vi "Sensado_mioelectrico_Final.vi"() -> ()   [LabVIEW 2010]
uses:
  <vilib>/express/express analysis/Spectral/XNode/ExpressSpectralMeasurementsBlockNode.xnode
  <vilib>/express/express analysis/Spectral/Block/exnSpectralBlock spectral measurements RMS poly.vi
  <vilib>/express/express analysis/Spectral/Block/exnSpectralBlock spectral measurements RMS WFM.vi
  <vilib>/measure/NI_MABase.lvlib
  <vilib>/express/express analysis/Spectral/Block/exnSpectralBlock spectral measurements power poly.vi
  <vilib>/express/express analysis/Spectral/Block/exnSpectralBlock spectral measurements power WFM.vi
  <vilib>/express/express analysis/Spectral/Block/exnSpectralBlock spectral measurements PSD poly.vi
  <vilib>/express/express analysis/Spectral/Block/exnSpectralBlock spectral measurements PSD WFM.vi
panel:
  in  "Lesion Off\nLesion On":bool
  out "Frecuencia normal":bool
  out "Persona Sana":bool
  out "Señal Anormal":bool
  out "Fatiga":bool
  out "Frecuencia promedio":dbl
  out "Voltaje RMS":dbl format="%0.2f"
  out "Tiempo s":u32
  out "SEMG Filtrada":waveform(dbl)(graph)
  out "FFT sin Filtrado":cluster{"f0":dbl, "df":dbl, "magnitude":dbl[]}(graph) caption="Filtered Signal"
  out "DDT Power Spectrum Density":cluster{"f0":dbl, "df":dbl, "magnitude":dbl[]}(graph) caption="Filtered Signal"
  out "Power Spectrum":cluster{"f0":dbl, "df":dbl, "magnitude":dbl[]}(graph) caption="Filtered Signal"
  out "FFT Filtrada":cluster{"f0":dbl, "df":dbl, "magnitude":dbl[]}(graph) caption="Filtered Signal"
  out "SEMG Bruto":waveform(dbl)(graph)
  in  "Stop":bool
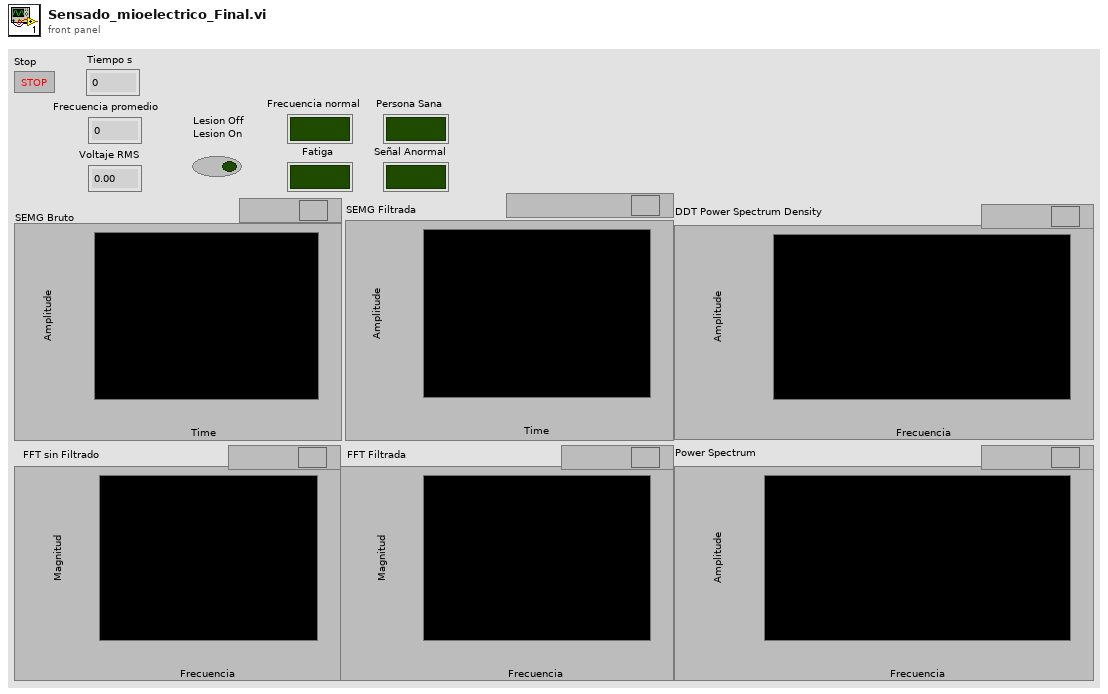
[diagram p1: front panel]
types:
  T1 = enum16{"Sine Wave", "Triangle Wave", "Square Wave", "Sawtooth Wave"}
  T2 = cluster{"averaging mode":u16, "weighting mode":u16, "number of averages":u32}
  T3 = cluster{"dB On (F)":bool, "unwrap phase (F)":bool, "convert to degree (F)":bool}
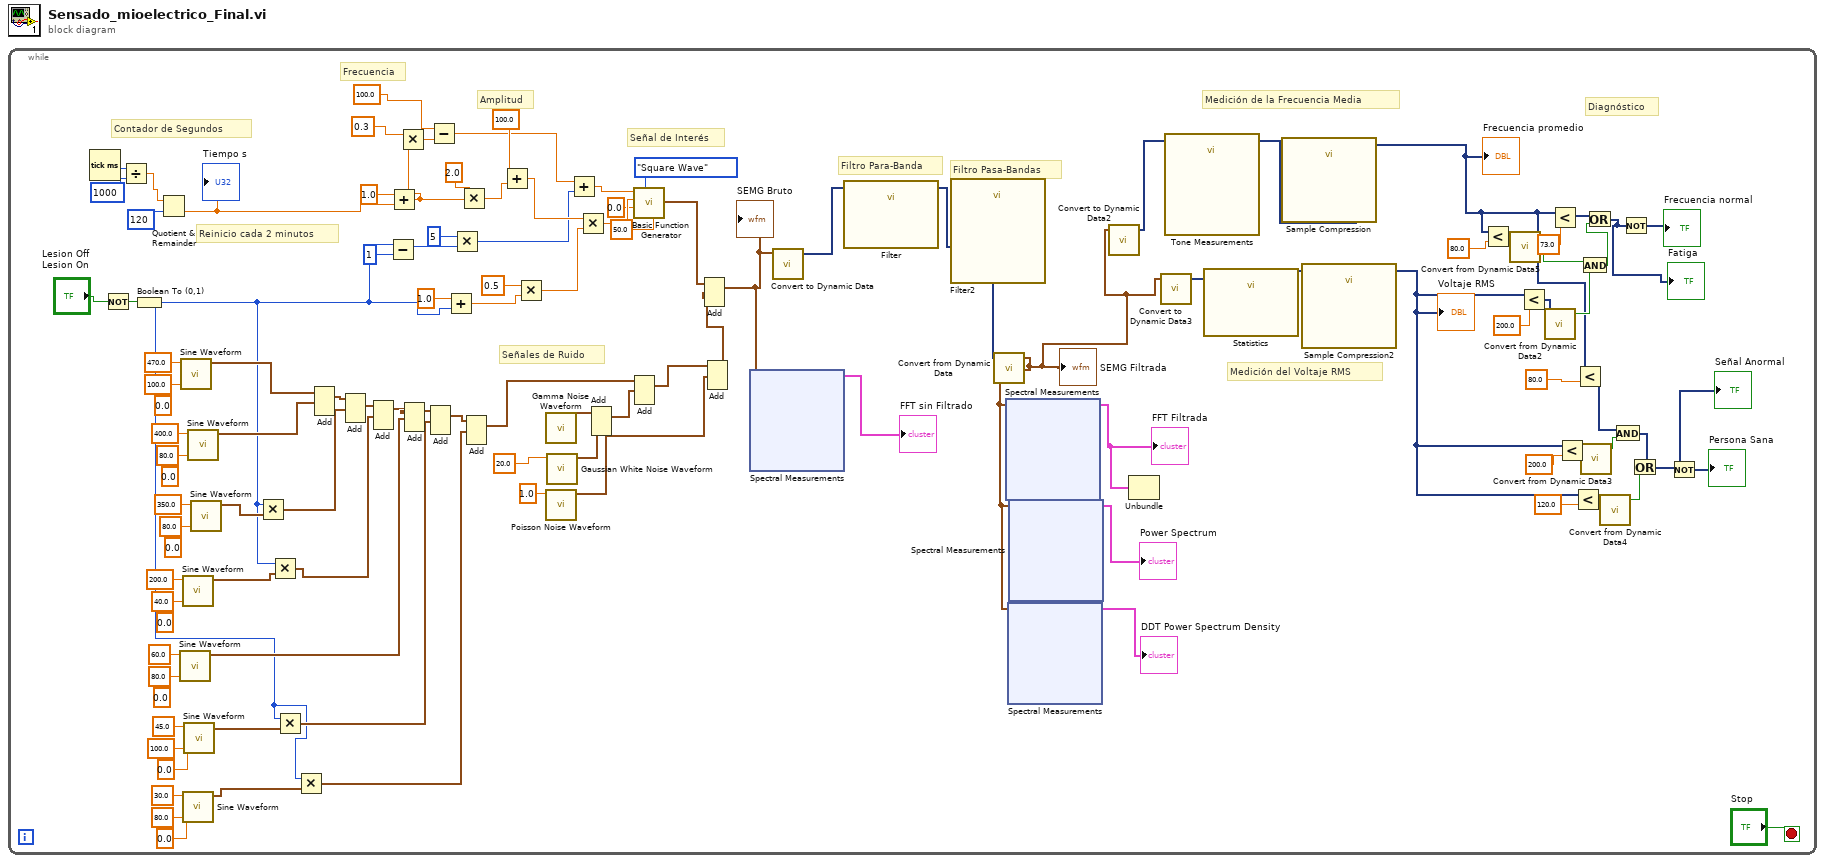
[diagram p0: block diagram]
diagram:
  n1 = while {
    stop <- "Stop" stop-if-true
    (unwired) 0.0 ("phase")
    (unwired) 0.0 ("phase")
    (unwired) 0.0 ("phase")
    (unwired) 0.0 ("phase")
    (unwired) 0.0 ("phase")
    # "Señal de Interés"
    # "Diagnóstico"
    # "Medición del Voltaje RMS"
    # "Medición de la Frecuencia Media"
    # "Filtro Pasa-Bandas"
    # "Filtro Para-Banda"
    # "Señales de Ruido"
    # "Reinicio cada 2 minutos"
    # "Contador de Segundos"
    # "Amplitud"
    # "Frecuencia"
    n2 = Tick Count (ms)() -> (millisecond timer value=w69:u32)
    n3 = Not(x="Lesion Off\nLesion On") -> (.not. x?=w37:bool)
    n4 = Divide(x=w69, y=u32 1000) -> (x/y=w67:dbl)
    n5 = Boolean To (0,1)(Boolean=w37) -> (0, 1=w17:i16)
    n6 = Quotient & Remainder(x=w67, y=u32 120) -> (x-y*floor(x/y)=w66:dbl)  [unwired: 1 out]
    "Tiempo s" <- w66
    n7 = call <vilib>:"Sine Waveform.vi"("amplitude"=80.0, "frequency"=60.0) -> ("signal out"=w71:waveform(dbl))  [unwired: 8 in, 1 out]
    n8 = call <vilib>:"Sine Waveform.vi"("amplitude"=100.0, "frequency"=470.0) -> ("signal out"=w79:waveform(dbl))  [unwired: 8 in, 1 out]
    n9 = call <vilib>:"Sine Waveform.vi"("amplitude"=40.0, "frequency"=200.0) -> ("signal out"=w28:waveform(dbl))  [unwired: 8 in, 1 out]
    n10 = call <vilib>:"Sine Waveform.vi"("phase"=0.0, "amplitude"=80.0, "frequency"=30.0) -> ("signal out"=w42:waveform(dbl))  [unwired: 7 in, 1 out]
    n11 = call <vilib>:"Sine Waveform.vi"("phase"=0.0, "amplitude"=100.0, "frequency"=45.0) -> ("signal out"=w41:waveform(dbl))  [unwired: 7 in, 1 out]
    n12 = call <vilib>:"Sine Waveform.vi"("amplitude"=80.0, "frequency"=400.0) -> ("signal out"=w78:waveform(dbl))  [unwired: 8 in, 1 out]
    n13 = call <vilib>:"Sine Waveform.vi"("amplitude"=80.0, "frequency"=350.0) -> ("signal out"=w29:waveform(dbl))  [unwired: 8 in, 1 out]
    n14 = Multiply(x=w17, y=w29) -> (x*y=w31:waveform(dbl))
    n15 = Multiply(x=w17, y=w28) -> (x*y=w30:waveform(dbl))
    n16 = Multiply(x=w17, y=w41) -> (x*y=w40:waveform(dbl))
    n17 = Multiply(x=w17, y=w42) -> (x*y=w39:waveform(dbl))
    n18 = Add(1:w78, 2:w79) -> (0:w77:waveform(dbl))  [unwired: 1 in, 1 out]
    n19 = Add(1:w31, 2:w77) -> (0:w73:waveform(dbl))  [unwired: 1 in, 1 out]
    n20 = Add(1:w30, 2:w73) -> (0:w72:waveform(dbl))  [unwired: 1 in, 1 out]
    n21 = Subtract(x=w17, y=i16 1) -> (x-y=w13:i16)
    n22 = Add(x=1.0, y=w66) -> (x+y=w62:dbl)
    n23 = Multiply(x=0.3, y=w62) -> (x*y=w60:dbl)
    n24 = Add(1:w71, 2:w72) -> (0:w84:waveform(dbl))  [unwired: 1 in, 1 out]
    n25 = Add(1:w40, 2:w84) -> (0:w88:waveform(dbl))  [unwired: 1 in, 1 out]
    n26 = Subtract(x=100.0, y=w60) -> (x-y=w14:dbl)
    n27 = Add(x=1.0, y=w17) -> (x+y=w36:dbl)
    n28 = Multiply(x=i16 5, y=w13) -> (x*y=w11:i16)
    n29 = Multiply(x=2.0, y=w62) -> (x*y=w63:dbl)
    n30 = Add(1:w39, 2:w88) -> (0:w91:waveform(dbl))  [unwired: 1 in, 1 out]
    n31 = Add(x=100.0, y=w63) -> (x+y=w34:dbl)
    n32 = Multiply(x=0.5, y=w36) -> (x*y=w33:dbl)
    n33 = call <vilib>:"Gamma Noise Waveform.vi"() -> ("signal out"=w104:waveform(dbl))  [unwired: 10 in, 1 out]
    n34 = call <vilib>:"Poisson Noise Waveform.vi"("mean"=1.0) -> ("signal out"=w101:waveform(dbl))  [unwired: 9 in, 1 out]
    n35 = call <vilib>:"Gaussian White Noise Waveform.vi"("standard deviation"=20.0) -> ("signal out"=w103:waveform(dbl))  [unwired: 9 in, 1 out]
    n36 = Add(x=w14, y=w11) -> (x+y=w15:dbl)
    n37 = Multiply(x=w34, y=w33) -> (x*y=w32:dbl)
    n38 = Add(1:w103, 2:w104) -> (0:w102:waveform(dbl))  [unwired: 1 in, 1 out]
    n39 = Add(1:w102, 2:w91) -> (0:w100:waveform(dbl))  [unwired: 1 in, 1 out]
    n40 = call <vilib>:"Basic Function Generator.vi"("square wave duty cycle (%)"=50.0, "signal type"=T1."Square Wave", "phase"=0.0, "amplitude"=w32, "frequency"=w15) -> ("signal out"=w105:waveform(dbl))  [unwired: 4 in, 2 out]
    n41 = Add(1:w101, 2:w100) -> (0:w99:waveform(dbl))  [unwired: 1 in, 1 out]
    n42 = Add(1:w99, 2:w105) -> (0:w44:waveform(dbl))  [unwired: 1 in, 1 out]
    "SEMG Bruto" <- w44
    n43 = xnode "Spectral Measurements"("Signals"=w44) -> ("FFT - (RMS)"=→"FFT sin Filtrado":cluster{"f0":dbl, "df":dbl, "magnitude":dbl[]})  [unwired: 1 in, 2 out]
    n44 = call "Convert to Dynamic Data"("Waveform"=w44) -> ("Dynamic Data Type"=w106:dynamicdata)  [unwired: 3 in]
    n45 = call "Filter"("Signal"=w106) -> ("Filtered Signal"=w97:dynamicdata)  [unwired: 9 in, 1 out]
    n46 = call "Filter2"("Signal"=w97) -> ("Filtered Signal"=w96:dynamicdata)  [unwired: 9 in, 1 out]
    n47 = call "Convert from Dynamic Data"("Dynamic Data Type"=w96) -> ("Waveform"=w52:waveform(dbl))  [unwired: 3 in]
    "SEMG Filtrada" <- w52
    n48 = xnode "Spectral Measurements"("Signals"=w52) -> ("FFT - (RMS)"=w59:cluster{"f0":dbl, "df":dbl, "magnitude":dbl[]})  [unwired: 1 in, 2 out]
    "FFT Filtrada" <- w59
    n49 = xnode "Spectral Measurements"("Signals"=w52) -> ("PSD"=→"DDT Power Spectrum Density":cluster{"f0":dbl, "df":dbl, "magnitude":dbl[]})  [unwired: 1 in, 1 out]
    n50 = xnode "Spectral Measurements"("Signals"=w52) -> ("Power Spectrum"=→"Power Spectrum":cluster{"f0":dbl, "df":dbl, "magnitude":dbl[]})  [unwired: 1 in, 1 out]
    n51 = call "Convert to Dynamic Data2"("Waveform"=w52) -> ("Dynamic Data Type"=w58:dynamicdata)  [unwired: 3 in]
    n52 = Unbundle(w59) -> ()  [unwired: 3 out]
    n53 = call "Convert to Dynamic Data3"("Waveform"=w52) -> ("Dynamic Data Type"=w51:dynamicdata)  [unwired: 3 in]
    n54 = call "Tone Measurements"("Signals"=w58) -> ("Frequency"=w57:dynamicdata)  [unwired: 9 in, 1 out]
    n55 = call "Statistics"("Signals"=w51) -> ("RMS"=w48:dynamicdata)  [unwired: 25 in, 1 out]
    n56 = call "Sample Compression"("Signals"=w57) -> ("Mean"=w3:dynamicdata)  [unwired: 8 in, 2 out]
    "Frecuencia promedio" <- w3
    n57 = call "Sample Compression2"("Signals"=w48) -> ("Mean"=w8:dynamicdata)  [unwired: 8 in, 2 out]
    "Voltaje RMS" <- w8
    n58 = Less?(x=w3, y=80.0) -> (x < y?=w2:dynamicdata)
    n59 = call "Convert from Dynamic Data5"("Dynamic Data Type"=w2) -> ("Scalar"=w1:bool)  [unwired: 3 in]
    n60 = Less?(x=w8, y=200.0) -> (x < y?=w6:dynamicdata)
    n61 = call "Convert from Dynamic Data2"("Dynamic Data Type"=w6) -> ("Scalar"=w50:bool)  [unwired: 3 in]
    n62 = Less?(x=w3, y=73.0) -> (x < y?=w9:dynamicdata)
    n63 = Less?(x=w8, y=200.0) -> (x < y?=w49:dynamicdata)
    n64 = Less?(x=w8, y=120.0) -> (x < y?=w24:dynamicdata)
    n65 = Less?(x=w3, y=80.0) -> (x < y?=w46:dynamicdata)
    n66 = And(x=w1, y=w50) -> (x .and. y?=w5:bool)
    n67 = call "Convert from Dynamic Data3"("Dynamic Data Type"=w49) -> ("Scalar"=w45:bool)  [unwired: 3 in]
    n68 = Or(x=w9, y=w5) -> (x .or. y?=w10:dynamicdata)
    "Fatiga" <- w10
    n69 = call "Convert from Dynamic Data4"("Dynamic Data Type"=w24) -> ("Scalar"=w25:bool)  [unwired: 3 in]
    n70 = And(x=w46, y=w45) -> (x .and. y?=w26:dynamicdata)
    n71 = Not(x=w10) -> (.not. x?=→"Frecuencia normal":dynamicdata)
    n72 = Or(x=w26, y=w25) -> (x .or. y?=w27:dynamicdata)
    "Señal Anormal" <- w27
    n73 = Not(x=w27) -> (.not. x?=→"Persona Sana":dynamicdata)
  }
